vi "实时数据参数入列队.vi"(11 "实时数据参数选择框":T1={"水样测量数据"=FALSE, "零点核查数据"=TRUE, "跨度核查数据"=TRUE, "加标回收数据"=TRUE, "平行样数据"=FALSE, "标样核查"=TRUE, "集成干预测试"=TRUE}) -> (0 "错误输出":errorcluster)   [LabVIEW 2016, in "数据传输系统.lvlib"]
panel:
  out "数组":string[](array[string])
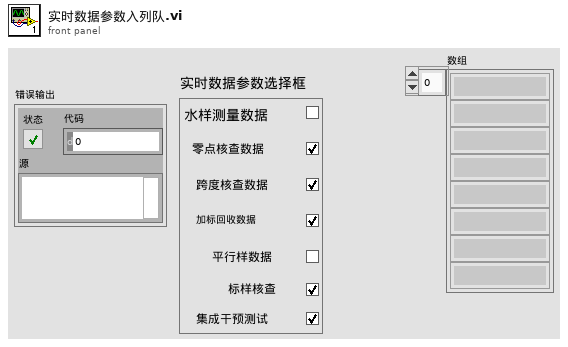
[diagram p1: front panel]
types:
  T1 = cluster{"水样测量数据":bool, "零点核查数据":bool, "跨度核查数据":bool, "加标回收数据":bool, "平行样数据":bool, "标样核查":bool, "集成干预测试":bool}
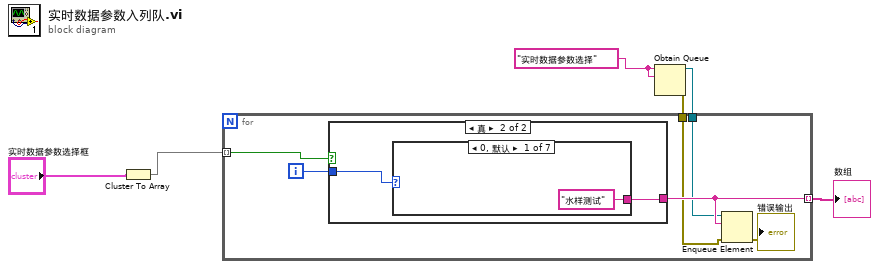
[diagram p0: block diagram]
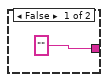
[diagram p2: hidden frame]
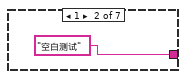
[diagram p3: hidden frame]
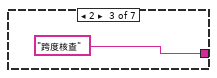
[diagram p4: hidden frame]
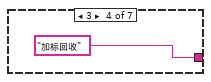
[diagram p5: hidden frame]
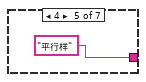
[diagram p6: hidden frame]
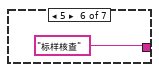
[diagram p7: hidden frame]
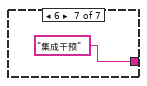
[diagram p8: hidden frame]
diagram:
  w4 = "实时数据参数选择" ("名称（未命名）")
  n1 = Cluster To Array(cluster="实时数据参数选择框") -> (array=w1:bool[])
  n2 = Obtain Queue(name (unnamed)=w4, element data type=w4) -> (queue out=w5:refnum<queue>, error out=w3:errorcluster)  [unwired: 3 in, 1 out]
  n3 = for {
    tunnel: w1 -> [w12] mode=indexing
    tunnel: [w10] -> w6 mode=indexing
    tunnel: w5 -> [w9]
    tunnel: w3 -> [w8]
    i -> [w11]
    n4 = case shown="真" w12 {
      tunnel: w11 -> [_ w15]
      tunnel: ["" ("Label.Text") w14] -> w10
      frame False {
      }
      frame True {
        n5 = case shown="0, 默认" w15 {
          tunnel: ["水样测试" ("Label.Text") "空白测试" ("Label.Text") "跨度核查" ("Label.Text") "加标回收" ("Label.Text") "平行样" ("Label.Text") "标样核查" ("Label.Text") "集成干预" ("Label.Text")] -> w14
          frame 0, Default {
          }
          frame 1 {
          }
          frame 2 {
          }
          frame 3 {
          }
          frame 4 {
          }
          frame 5 {
          }
          frame 6 {
          }
        }
      }
    }
    n6 = Enqueue Element(queue=w9, element=w10, error in (no error)=w8) -> (error out=→"错误输出":errorcluster)  [unwired: 1 in, 2 out]
  }
  "数组" <- w6
